vi "ExitApplication Event Callback.vi"(4 "GUI.lvlib:Auto UI.lvlib:Auto UI.lvclass":refnum<class "Auto UI.lvclass">, 6 "CtlRef":refnum<k7>, 7 "Event common data":cluster{"Source":i32, "Type":u32, "Time":u32}) -> ()   [LabVIEW 2023, in "GUI.lvlib" / "Auto UI.lvlib" / "Auto UI.lvclass"]
uses:
  Auto UI.lvclass
  Auto UI.lvclass/Auto UI.ctl
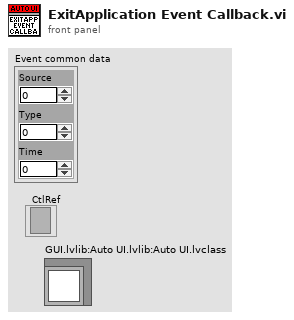
[diagram p1: front panel]
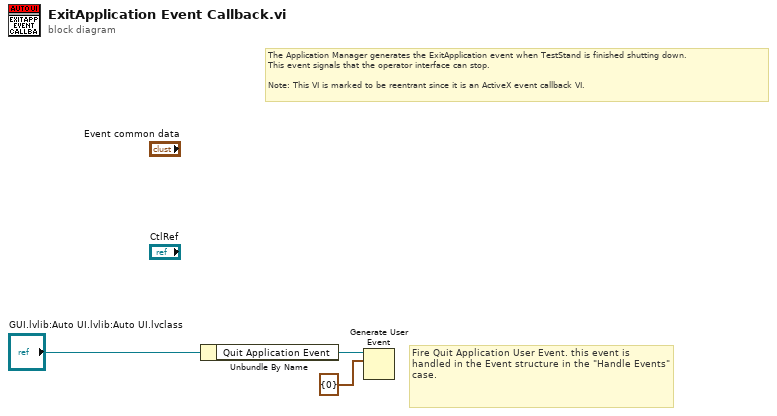
[diagram p0: block diagram]
diagram:
  # "Fire Quit Application User Event. this event is handled in the Event structure in the \"Handle Events\" case."
  # "The Application Manager generates the ExitApplication event when TestStand is finished shutting down.\nThis event signals that the operator interface can stop.\n\nNote: This VI is marked to be reentrant since it is an ActiveX event callback VI."
  n1 = Unbundle By Name("GUI.lvlib:Auto UI.lvlib:Auto UI.lvclass") -> ("Quit Application Event"=w2:refnum<user-event>)
  n2 = Generate User Event(user event=w2, event data cluster=cluster{i32} {0}) -> ()  [unwired: 2 in, 2 out]
